vi "AK Komm_ALT.vi"(6 "Aktionen_ALT":T2=enum."initialisieren", 11 "Daten":string[](array[string])) -> (0 "Verfügbare Gase":string[][](array[string]), 1 "Empfangsdaten":string[](array[string]), 2 "Error":T1, 3 "Status":string, 4 "Störung Kommunikation":bool)   [LabVIEW 2020, in "Linearisierung v2.lvlib" / "Gasteiler.lvlib" / "AK Komm Gasteiler.lvlib" / "Alter Gasteiler.lvlib"]
uses:
  Alter Gasteiler.lvlib
  Aktionen AK Komm_ALT.ctl
  Gasteiler Fehler.ctl
  Aktionen FGV Gasteiler Daten.ctl
  AK Komm Gasteiler.lvlib
  Gasteiler.lvlib
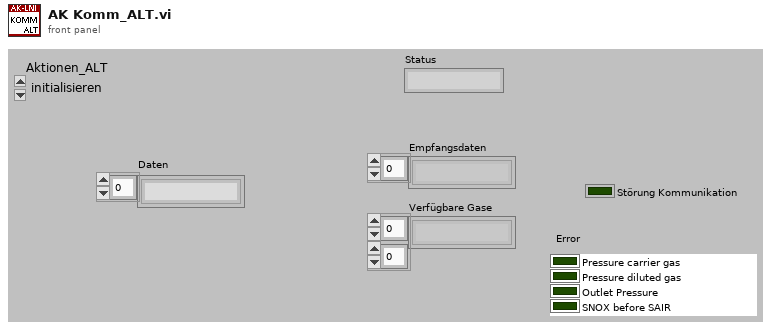
[diagram p1: front panel]
types:
  T1 = typedef "Linearisierung v2.lvlib/Gasteiler.lvlib/Gasteiler Fehler.ctl" = cluster{"Pressure carrier gas":bool, "Pressure diluted gas":bool, "Outlet Pressure":bool, "SNOX before SAIR":bool}
  T2 = typedef "Linearisierung v2.lvlib/Gasteiler.lvlib/AK Komm Gasteiler.lvlib/Alter Gasteiler.lvlib/Aktionen AK Komm_ALT.ctl" = enum16{"lesen", "initialisieren", "beenden", "SRES", "STBY", "SREM", "SMAN", "SLIN", "SLCH", "SLST", "SSPL", "AGAT", "ALST", "ASTZ", "ASTF", "AGAK", "EGAK"}
  T3 = typedef "Linearisierung v2.lvlib/Gasteiler.lvlib/Aktionen FGV Gasteiler Daten.ctl" = enum16{"lesen", "Gasteiler Daten", "Seriellen Param.", "MB-Endwert", "laden", "speichern", "Anforderung", "TCP", "Aufzeichnung Start"}
  T4 = typedef "AK-Schnittstelle.lvlib/AK Seriell.lvlib/Serielle Parameter.ctl" = cluster{"VISA resource name":refnum<visa-resource-name>, "baud rate":u32, "data bits":u16, "parity":u16, "stop bits":u16, "flow control":u16}
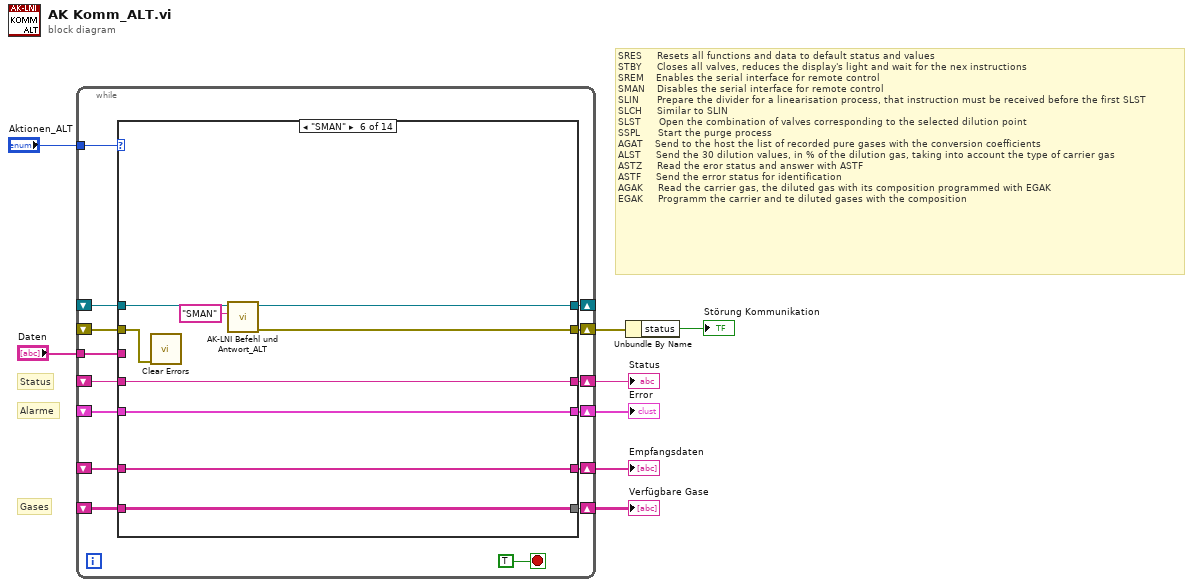
[diagram p0: block diagram]
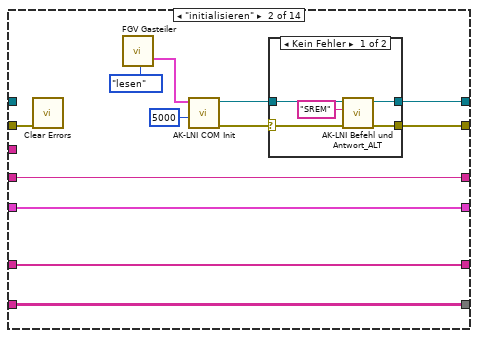
[diagram p3: hidden frame]
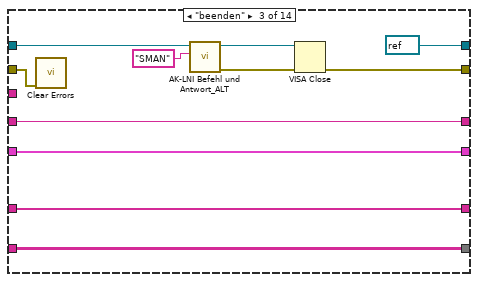
[diagram p5: hidden frame]
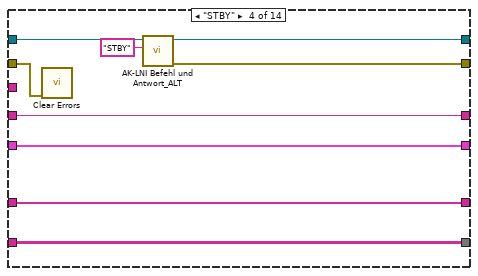
[diagram p6: hidden frame]
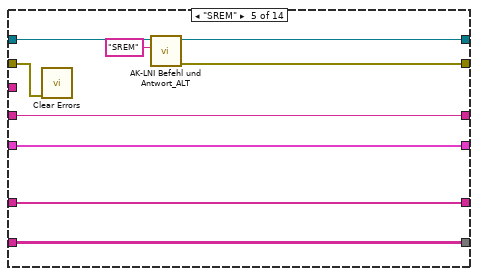
[diagram p7: hidden frame]
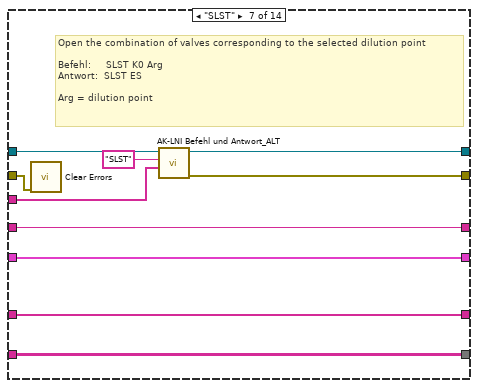
[diagram p8: hidden frame]
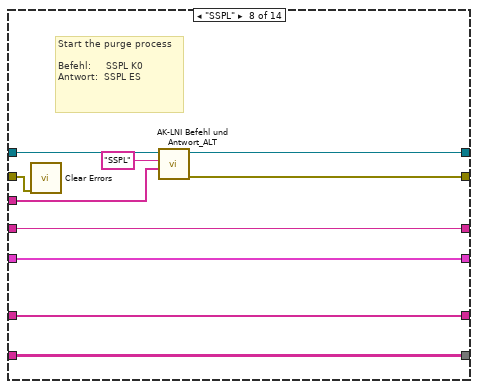
[diagram p9: hidden frame]
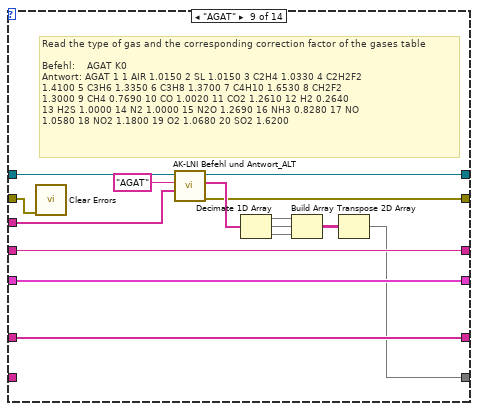
[diagram p10: hidden frame]
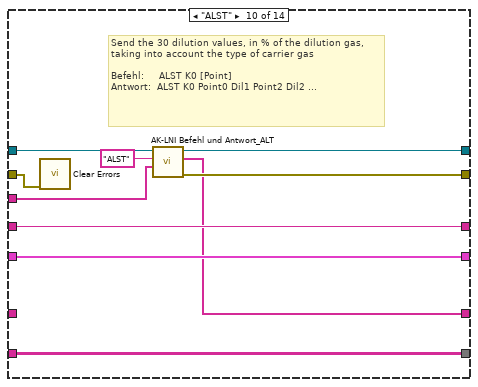
[diagram p11: hidden frame]
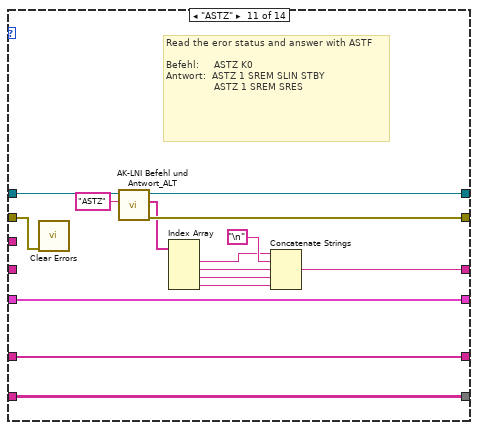
[diagram p12: hidden frame]
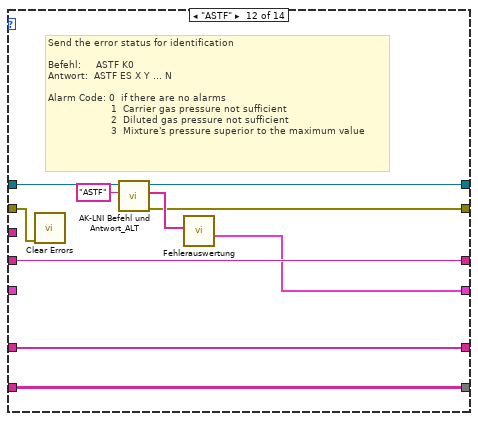
[diagram p13: hidden frame]
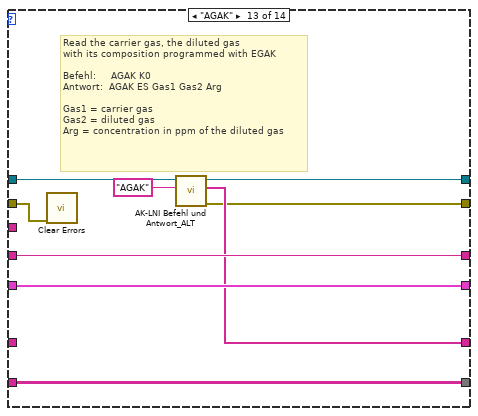
[diagram p14: hidden frame]
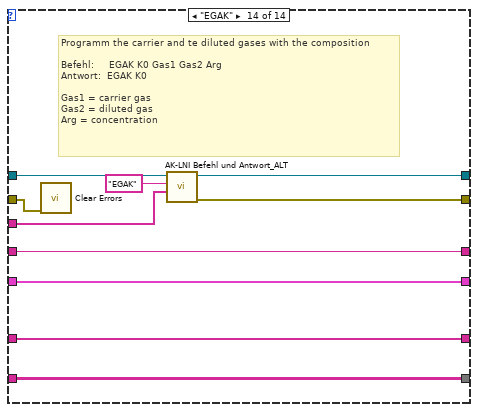
[diagram p15: hidden frame]
diagram:
  # "SRES     Resets all functions and data to default status and values\nSTBY     Closes all valves, reduces the display's light and wait for the nex instructions\nSREM    Enables the serial interface for remote control\nSMAN    Disables the serial interface for remote control\nSLIN      Prepare the divider for a linearisation process, that instruction must be received before the first SLST\nSLCH     Similar to SLIN\nSLST      Open the combination of valves corresponding to the selected dilution point\nSSPL      Start the purge process \nAGAT    Send to the host the list of recorded pure gases with the conversion coefficients\nALST     Send the 30 dilution values, in % of the dilution gas, taking into account the type of carrier gas\nASTZ     Read the eror status and answer with ASTF\nASTF     Send the error status for identification\nAGAK     Read the carrier gas, the diluted gas with its composition programmed with EGAK\nEGAK     Programm the carrier and te diluted gases with the composition"
  # "Gases"
  # "Status"
  # "Alarme"
  n1 = while {
    tunnel: "Aktionen_ALT" -> [w22]
    shift-right: [w21] -> _
    shift-left: _ -> [w20]
    shift-right: [w19] -> w3
    shift-left: _ -> [w18]
    shift-right: [w16] -> w6
    shift-left: _ -> [w17]
    tunnel: "Daten" -> [w15]
    shift-right: [w14] -> w4
    shift-left: _ -> [w13]
    shift-right: [w12] -> w5
    shift-left: _ -> [w11]
    shift-right: [w10] -> w2
    shift-left: _ -> [w9]
    stop <- TRUE stop-if-true
    n2 = case shown="\"SMAN\"" w22 {
      tunnel: [w28 w34 refnum<visa-resource-name> refnum ("VISA resource name") w66 w75 w84 w94 w104 w119 w129 w144 w154 w163 w173] -> w21
      tunnel: w20 -> [w28 _ w52 w68 w77 w86 w96 w106 w121 w131 w146 w156 w165 w175]
      tunnel: [w29 w40 w58 w65 w74 w83 w93 w103 w118 w128 w143 w148 w162 w172] -> w19
      tunnel: w18 -> [w29 w40 w58 w65 w74 w83 w93 w103 w118 w128 w143 _ w162 w172]
      tunnel: w17 -> [w26 w39 w57 w64 w73 w82 w91 w101 w116 w126 _ w152 w161 w170]
      tunnel: [w26 w39 w57 w64 w73 w82 w91 w101 w116 w126 w134 w152 w161 w170] -> w16
      tunnel: w15 -> [_ _ _ _ _ _ w92 w102 w117 w127 _ _ _ w171]
      tunnel: [w25 w37 w55 w62 w71 w80 w89 w99 w108 w125 w142 w150 w160 w169] -> w14
      tunnel: w13 -> [w25 w37 w55 w62 w71 w80 w89 w99 _ w125 w142 w150 w160 w169]
      tunnel: [w27 w38 w56 w63 w72 w81 w90 w100 w112 w122 w132 w151 w159 w168] -> w12
      tunnel: w11 -> [w27 w38 w56 w63 w72 w81 w90 w100 w112 _ w132 w151 _ w168]
      tunnel: [w24 w32 w54 w61 w70 w79 w88 w98 w111 w124 w141 w149 w158 w167] -> w10
      tunnel: w9 -> [w24 w36 w53 w60 w69 w78 w87 w97 w110 w123 w140 w147 w157 w166]
      frame "lesen", Default {
      }
      frame "initialisieren" {
        n3 = call <vilib>:"Clear Errors.vi"("error in (no error)"=w36) -> ()  [unwired: 5 in, 2 out]
        n4 = call "FGV Gasteiler.vi"("Aktionen"=Aktionen_FGV_Gasteiler_Daten."lesen") -> ("Serielle Parameter"=w30:T4)  [unwired: 11 in, 7 out]
        n5 = call "AK-LNI COM Init.vi"("TimeOut (ms)"=u32 5000, "Schnittstelle"=w30) -> ("error out"=w33:errorcluster, "VISA resource name"=w35:refnum<visa-resource-name>)  [unwired: 8 in]
        n6 = case shown="Kein Fehler" w33 {
          selector: w33 -> [w43 w47]
          tunnel: w35 -> [w45 w48]
          tunnel: [w44 w48] -> w34
          tunnel: [w42 w47] -> w32
          frame No Error {
            n7 = call "AK-LNI Befehl und Antwort_ALT.vi"("Fehler (Eingang)"=w43, "Befehl (4 Zeichen)"="SREM", "VISA resource name"=w45) -> ("Fehler (Ausgang)"=w42:errorcluster, "VISA resource name out"=w44:refnum<visa-resource-name>)  [unwired: 3 in, 4 out]
          }
          frame Error {
          }
        }
      }
      frame "beenden" {
        n8 = call <vilib>:"Clear Errors.vi"("error in (no error)"=w53) -> ()  [unwired: 5 in, 2 out]
        n9 = call "AK-LNI Befehl und Antwort_ALT.vi"("Befehl (4 Zeichen)"="SMAN", "VISA resource name"=w52) -> ("Fehler (Ausgang)"=w49:errorcluster, "VISA resource name out"=w50:refnum<visa-resource-name>)  [unwired: 4 in, 4 out]
        n10 = VISA Close(VISA resource name=w50, error in (no error)=w49) -> (error out=w54:errorcluster)
      }
      frame "STBY" {
        n11 = call <vilib>:"Clear Errors.vi"("error in (no error)"=w60) -> ()  [unwired: 5 in, 2 out]
        n12 = call "AK-LNI Befehl und Antwort_ALT.vi"("Befehl (4 Zeichen)"="STBY", "VISA resource name"=w68) -> ("Fehler (Ausgang)"=w61:errorcluster, "VISA resource name out"=w66:refnum<visa-resource-name>)  [unwired: 4 in, 4 out]
      }
      frame "SREM" {
        n13 = call <vilib>:"Clear Errors.vi"("error in (no error)"=w69) -> ()  [unwired: 5 in, 2 out]
        n14 = call "AK-LNI Befehl und Antwort_ALT.vi"("Befehl (4 Zeichen)"="SREM", "VISA resource name"=w77) -> ("Fehler (Ausgang)"=w70:errorcluster, "VISA resource name out"=w75:refnum<visa-resource-name>)  [unwired: 4 in, 4 out]
      }
      frame "SMAN" {
        n15 = call <vilib>:"Clear Errors.vi"("error in (no error)"=w78) -> ()  [unwired: 5 in, 2 out]
        n16 = call "AK-LNI Befehl und Antwort_ALT.vi"("Befehl (4 Zeichen)"="SMAN", "VISA resource name"=w86) -> ("Fehler (Ausgang)"=w79:errorcluster, "VISA resource name out"=w84:refnum<visa-resource-name>)  [unwired: 4 in, 4 out]
      }
      frame "SLST" {
        # "Open the combination of valves corresponding to the selected dilution point\n\nBefehl:     SLST K0 Arg\nAntwort:  SLST ES\n\nArg = dilution point"
        n17 = call <vilib>:"Clear Errors.vi"("error in (no error)"=w87) -> ()  [unwired: 5 in, 2 out]
        n18 = call "AK-LNI Befehl und Antwort_ALT.vi"("Sendedaten"=w92, "Befehl (4 Zeichen)"="SLST", "VISA resource name"=w96) -> ("Fehler (Ausgang)"=w88:errorcluster, "VISA resource name out"=w94:refnum<visa-resource-name>)  [unwired: 3 in, 4 out]
      }
      frame "SSPL" {
        # "Start the purge process \n\nBefehl:     SSPL K0 \nAntwort:  SSPL ES"
        n19 = call <vilib>:"Clear Errors.vi"("error in (no error)"=w97) -> ()  [unwired: 5 in, 2 out]
        n20 = call "AK-LNI Befehl und Antwort_ALT.vi"("Sendedaten"=w102, "Befehl (4 Zeichen)"="SSPL", "VISA resource name"=w106) -> ("Fehler (Ausgang)"=w98:errorcluster, "VISA resource name out"=w104:refnum<visa-resource-name>)  [unwired: 3 in, 4 out]
      }
      frame "AGAT" {
        # "Read the type of gas and the corresponding correction factor of the gases table\n\nBefehl:    AGAT K0\nAntwort: AGAT 1 1 AIR 1.0150 2 SL 1.0150 3 C2H4 1.0330 4 C2H2F2\n1.4100 5 C3H6 1.3350 6 C3H8 1.3700 7 C4H10 1.6530 8 CH2F2\n1.3000 9 CH4 0.7690 10 CO 1.0020 11 CO2 1.2610 12 H2 0.2640\n13 H2S 1.0000 14 N2 1.0000 15 N2O 1.2690 16 NH3 0.8280 17 NO\n1.0580 18 NO2 1.1800 19 O2 1.0680 20 SO2 1.6200"
        n21 = call <vilib>:"Clear Errors.vi"("error in (no error)"=w110) -> ()  [unwired: 5 in, 2 out]
        n22 = call "AK-LNI Befehl und Antwort_ALT.vi"("Sendedaten"=w117, "Befehl (4 Zeichen)"="AGAT", "VISA resource name"=w121) -> ("Fehler (Ausgang)"=w111:errorcluster, "Empfangsdaten"=w115:string[], "VISA resource name out"=w119:refnum<visa-resource-name>)  [unwired: 3 in, 3 out]
        n23 = Decimate 1D Array(w115) -> (w114:string[], w113:string[], w107:string[])
        n24 = Build Array(w114, w113, w107) -> (w109:string[][])
        n25 = Transpose 2D Array(2D array=w109) -> (transposed array=w108:string[][])
      }
      frame "ALST" {
        # "Send the 30 dilution values, in % of the dilution gas,\ntaking into account the type of carrier gas\n\nBefehl:     ALST K0 [Point]\nAntwort:  ALST K0 Point0 Dil1 Point2 Dil2 ..."
        n26 = call <vilib>:"Clear Errors.vi"("error in (no error)"=w123) -> ()  [unwired: 5 in, 2 out]
        n27 = call "AK-LNI Befehl und Antwort_ALT.vi"("Sendedaten"=w127, "Befehl (4 Zeichen)"="ALST", "VISA resource name"=w131) -> ("Fehler (Ausgang)"=w124:errorcluster, "Empfangsdaten"=w122:string[], "VISA resource name out"=w129:refnum<visa-resource-name>)  [unwired: 3 in, 3 out]
      }
      frame "ASTZ" {
        # "Read the eror status and answer with ASTF\n\nBefehl:     ASTZ K0\nAntwort:  ASTZ 1 SREM SLIN STBY\n                ASTZ 1 SREM SRES"
        n28 = call <vilib>:"Clear Errors.vi"("error in (no error)"=w140) -> ()  [unwired: 5 in, 2 out]
        n29 = call "AK-LNI Befehl und Antwort_ALT.vi"("Befehl (4 Zeichen)"="ASTZ", "VISA resource name"=w146) -> ("Fehler (Ausgang)"=w141:errorcluster, "Empfangsdaten"=w133:string[], "VISA resource name out"=w144:refnum<visa-resource-name>)  [unwired: 4 in, 3 out]
        n30 = Index Array(array=w133) -> (element #1=w138:string, element #2=w137:string, element #3=w136:string, element #4=w135:string)  [unwired: 4 in]
        n31 = Concatenate Strings(w138, "\n", w137, w136, w135) -> (w134:string)
      }
      frame "ASTF" {
        # "Send the error status for identification\n\nBefehl:     ASTF K0\nAntwort:  ASTF ES X Y ... N\n\nAlarm Code: 0  if there are no alarms\n                     1  Carrier gas pressure not sufficient\n                     2  Diluted gas pressure not sufficient\n                     3  Mixture's pressure superior to the maximum value"
        n32 = call <vilib>:"Clear Errors.vi"("error in (no error)"=w147) -> ()  [unwired: 5 in, 2 out]
        n33 = call "AK-LNI Befehl und Antwort_ALT.vi"("Befehl (4 Zeichen)"="ASTF", "VISA resource name"=w156) -> ("Fehler (Ausgang)"=w149:errorcluster, "Empfangsdaten"=w153:string[], "VISA resource name out"=w154:refnum<visa-resource-name>)  [unwired: 4 in, 3 out]
        n34 = call "Fehlerauswertung.vi"("Empfangsdaten"=w153) -> ("Error"=w148:T1)  [unwired: 9 in, 1 out]
      }
      frame "AGAK" {
        # "Read the carrier gas, the diluted gas\nwith its composition programmed with EGAK\n\nBefehl:     AGAK K0\nAntwort:  AGAK ES Gas1 Gas2 Arg\n\nGas1 = carrier gas\nGas2 = diluted gas\nArg = concentration in ppm of the diluted gas"
        n35 = call <vilib>:"Clear Errors.vi"("error in (no error)"=w157) -> ()  [unwired: 5 in, 2 out]
        n36 = call "AK-LNI Befehl und Antwort_ALT.vi"("Befehl (4 Zeichen)"="AGAK", "VISA resource name"=w165) -> ("Fehler (Ausgang)"=w158:errorcluster, "Empfangsdaten"=w159:string[], "VISA resource name out"=w163:refnum<visa-resource-name>)  [unwired: 4 in, 3 out]
      }
      frame "EGAK" {
        # "Programm the carrier and te diluted gases with the composition\n\nBefehl:     EGAK K0 Gas1 Gas2 Arg\nAntwort:  EGAK K0\n\nGas1 = carrier gas\nGas2 = diluted gas\nArg = concentration"
        n37 = call <vilib>:"Clear Errors.vi"("error in (no error)"=w166) -> ()  [unwired: 5 in, 2 out]
        n38 = call "AK-LNI Befehl und Antwort_ALT.vi"("Sendedaten"=w171, "Befehl (4 Zeichen)"="EGAK", "VISA resource name"=w175) -> ("Fehler (Ausgang)"=w167:errorcluster, "VISA resource name out"=w173:refnum<visa-resource-name>)  [unwired: 3 in, 4 out]
      }
    }
  }
  "Status" <- w6
  "Empfangsdaten" <- w5
  "Verfügbare Gase" <- w4
  "Error" <- w3
  n39 = Unbundle By Name(w2) -> ("status"=→"Störung Kommunikation":bool)
